vi "AWS-S3-BucketSettings.vi"(0 "AWS-S3-API":refnum<class "AWS-S3-API.lvclass">, 5 "Bucket Name":string, 11 "error in":errorcluster) -> (4 "AWS-S3-API out":refnum<class "AWS-S3-API.lvclass">, 6 "Location":string, 8 "Versioning":enum16{"Unknown", "Off", "Enabled", "Suspended"}(ring), 10 "Log Target Bucket Name":string, 14 "Index Document":string, 15 "error out":errorcluster)   [LabVIEW 2012, in "AWS-S3-API.lvclass"]
uses:
  AWS-S3-API.lvclass
  C:/Users/Jack/repo/visualize/Dependencies/aws/AWS-SDK/AWSSDK.dll
  AWS-SDK/AWSSDK.dll
panel:
  # "Inputs"
  # "Outputs"
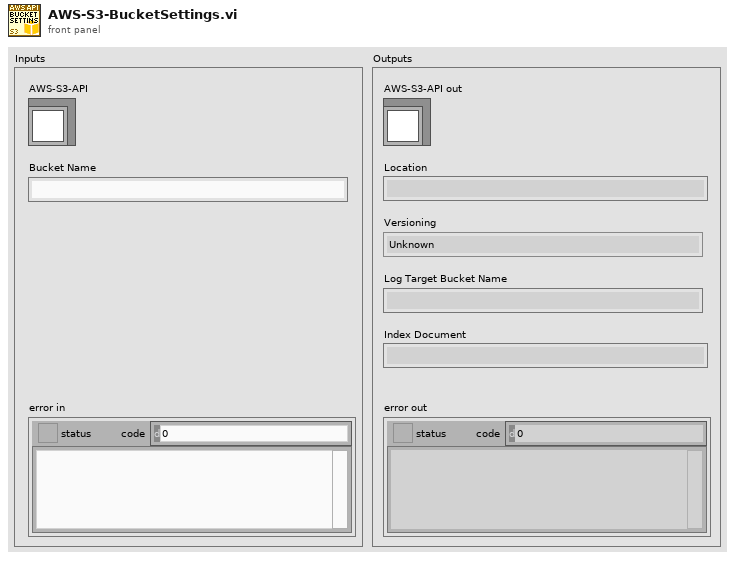
[diagram p1: front panel]
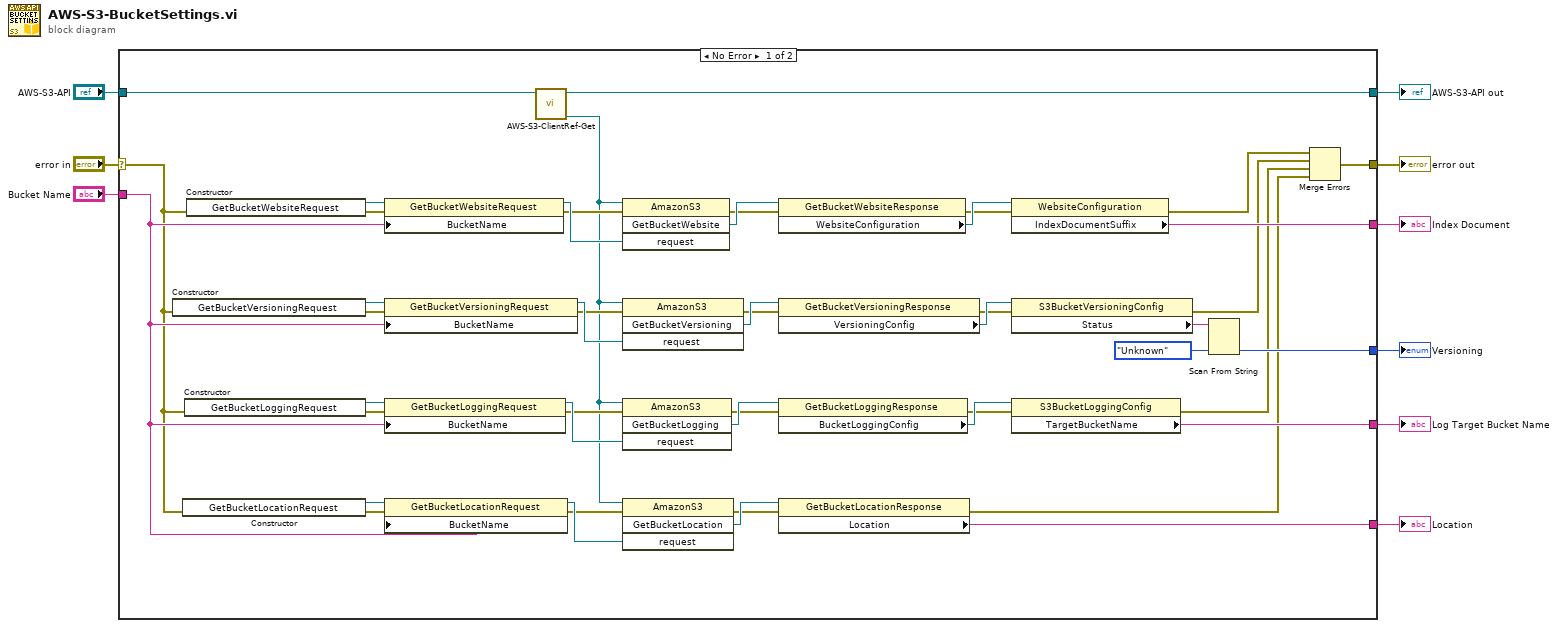
[diagram p0: block diagram]
diagram:
  n1 = case shown="No Error" "error in" {
    selector: "error in" -> [w30 w57]
    tunnel: [w14 w57] -> w9
    tunnel: [w10 w56] -> w7
    tunnel: "AWS-S3-API" -> [w11 w56]
    tunnel: [w52 _] -> w5
    tunnel: "Bucket Name" -> [w35 _]
    tunnel: [w45 _] -> w3
    tunnel: [w38 _] -> w2
    tunnel: [w31 _] -> w1
    frame No Error {
      n2 = constructor class="GetBucketVersioningRequest"(error in=w30) -> (reference out=w43:refnum<k24>, error out=w44:errorcluster)  [unwired: 2 in, 1 out]
      n3 = constructor class="GetBucketLocationRequest"(error in=w30) -> (reference out=w54:refnum<k24>, error out=w55:errorcluster)  [unwired: 2 in, 1 out]
      n4 = constructor class="GetBucketLoggingRequest"(error in=w30) -> (reference out=w50:refnum<k24>, error out=w49:errorcluster)  [unwired: 2 in, 1 out]
      n5 = constructor class="GetBucketWebsiteRequest"(error in=w30) -> (reference out=w37:refnum<k24>, error out=w36:errorcluster)  [unwired: 2 in, 1 out]
      n6 = property class="GetBucketWebsiteRequest"(reference=w37, error in=w36, "BucketName"=w35) -> (reference out=w34:refnum<k24>, error out=w25:errorcluster)
      n7 = property class="GetBucketVersioningRequest"(reference=w43, error in=w44, "BucketName"=w35) -> (reference out=w42:refnum<k24>, error out=w26:errorcluster)
      n8 = property class="GetBucketLoggingRequest"(reference=w50, error in=w49, "BucketName"=w35) -> (reference out=w48:refnum<k24>, error out=w27:errorcluster)
      n9 = property class="GetBucketLocationRequest"(reference=w54, error in=w55, "BucketName"=w35) -> (reference out=w51:refnum<k24>, error out=w28:errorcluster)
      n10 = call "AWS-S3-ClientRef-Get.vi"("AWS-S3-API"=w11) -> ("S3 Client ref"=w13:refnum<k24>, "AWS-S3-API out"=w10:refnum<class "AWS-S3-API.lvclass">)  [unwired: 9 in]
      n11 = invoke class="AmazonS3" method="GetBucketWebsite"(reference=w13, error in=w25, "request"=w34) -> (error out=w29:errorcluster, "GetBucketWebsite"=w33:refnum<k24>)  [unwired: 1 in, 2 out]
      n12 = invoke class="AmazonS3" method="GetBucketVersioning"(reference=w13, error in=w26, "request"=w42) -> (error out=w24:errorcluster, "GetBucketVersioning"=w40:refnum<k24>)  [unwired: 1 in, 2 out]
      n13 = invoke class="AmazonS3" method="GetBucketLogging"(reference=w13, error in=w27, "request"=w48) -> (error out=w23:errorcluster, "GetBucketLogging"=w47:refnum<k24>)  [unwired: 1 in, 2 out]
      n14 = invoke class="AmazonS3" method="GetBucketLocation"(reference=w13, error in=w28, "request"=w51) -> (error out=w22:errorcluster, "GetBucketLocation"=w53:refnum<k24>)  [unwired: 1 in, 2 out]
      n15 = property class="GetBucketWebsiteResponse"(reference=w33, error in=w29) -> (error out=w21:errorcluster, "WebsiteConfiguration"=w32:refnum<k24>)  [unwired: 1 out]
      n16 = property class="GetBucketVersioningResponse"(reference=w40, error in=w24) -> (error out=w20:errorcluster, "VersioningConfig"=w41:refnum<k24>)  [unwired: 1 out]
      n17 = property class="GetBucketLoggingResponse"(reference=w47, error in=w23) -> (error out=w19:errorcluster, "BucketLoggingConfig"=w46:refnum<k24>)  [unwired: 1 out]
      n18 = property class="GetBucketLocationResponse"(reference=w53, error in=w22) -> (error out=w15:errorcluster, "Location"=w52:string)  [unwired: 1 out]
      n19 = property class="WebsiteConfiguration"(reference=w32, error in=w21) -> (error out=w18:errorcluster, "IndexDocumentSuffix"=w31:string)  [unwired: 1 out]
      n20 = property class="S3BucketVersioningConfig"(reference=w41, error in=w20) -> (error out=w17:errorcluster, "Status"=w39:string)  [unwired: 1 out]
      n21 = property class="S3BucketLoggingConfig"(reference=w46, error in=w19) -> (error out=w16:errorcluster, "TargetBucketName"=w45:string)  [unwired: 1 out]
      n22 = Scan From String(input string=w39, default 1=enum16{"Unknown", "Off", "Enabled", "Suspended"}."Unknown" ("Versioning")) -> (output 1=w38:enum16{"Unknown", "Off", "Enabled", "Suspended"})  [unwired: 3 in, 3 out]
      n23 = Merge Errors(w18, w17, w16, w15) -> (w14:errorcluster)
    }
    frame Error {
    }
  }
  "error out" <- w9
  "AWS-S3-API out" <- w7
  "Versioning" <- w2
  "Log Target Bucket Name" <- w3
  "Index Document" <- w1
  "Location" <- w5
